vi "Update States.vi"(8 "error in (no error)":errorcluster, 11 "ATM Controller in":refnum<class "ATM Controller.lvclass">) -> (0 "error out":errorcluster, 3 "ATM Controller out":refnum<class "ATM Controller.lvclass">)   [LabVIEW 2019, in "ATM Controller.lvlib" / "ATM Controller.lvclass"]
uses:
  ATM Controller.lvclass
  ATM Controller Messages/Set State Msg/Set State Msg.lvclass
  <vilib>/ActorFramework/Actor/Actor.lvclass
  State -Enum.ctl
  ATM Controller Messages/Set ATM Message Msg/Set ATM Message Msg.lvclass
  Message Name.ctl
  Simulated User Console Actor/Simulated User Console Actor Messages/Enable Card Reader Msg/Enable Card Reader Msg.lvclass
  Simulated User Console Actor/Simulated User Console Actor Messages/Enable Keypad Msg/Enable Keypad Msg.lvclass
  Simulated User Console Actor/Simulated User Console Actor Messages/Enable Transaction Msg/Enable Transaction Msg.lvclass
  Simulated Display Console Actor/Simulated Display Console Actor Messages/Write Card Read Msg/Write Card Read Msg.lvclass
  Simulated Display Console Actor/Simulated Display Console Actor Messages/Write Current Transaction Msg/Write Current Transaction Msg.lvclass
  Simulated Sensor Interface Actor/Simulated Sensor Interface Actor Messages/Disable All Controls Msg/Disable All Controls Msg.lvclass
  Simulated User Console Actor/Simulated User Console Actor Messages/Write Card Reader Msg/Write Card Reader Msg.lvclass
  Simulated User Console Actor/Simulated User Console Actor Messages/Disable Terminate Session Msg/Disable Terminate Session Msg.lvclass
  Simulated Configuration Database Actor/Configuration Database Actor Messages/Read Record Msg/Read Record Msg.lvclass
  <vilib>/ActorFramework/Message Enqueuer/Message Enqueuer.lvclass
  Simulated Configuration Database Actor/Configuration Database Actor Messages/Write Record Msg/Write Record Msg.lvclass
  ATM Controller Messages/Set Timeout Msg/Set Timeout Msg.lvclass
  Simulated User Console Actor/Simulated User Console Actor/Transactions -Cluster.ctl
  Simulated User Console Actor/Simulated User Console Actor/Simulated User Console Actor.lvclass
  Simulated User Console Actor/Simulated User Console Actor Messages/Enable New Transaction Msg/Enable New Transaction Msg.lvclass
  C:/Program Files (x86)/National Instruments/LabVIEW 2019/vi.lib/ActorFramework/Actor/Actor.lvclass
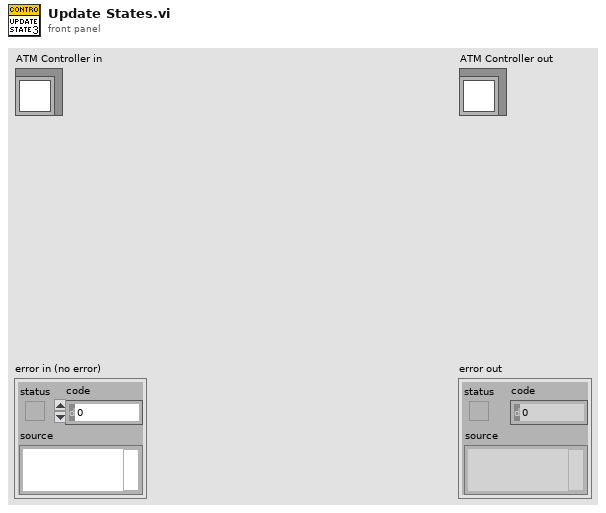
[diagram p1: front panel]
types:
  T1 = enum8{"Enabled", "Disabled", "Disabled and Grayed Out"}
  T2 = typedef "ATM Controller.lvlib/ATM Controller.lvclass/Message Name.ctl" = enum16{"Welcome", "Login", "Idle", "Invalid Login", "Terminate Session", "Deposit", "Withdrawal", "Fast Cash $50", "Withdrawal Failed", "Balance Inquiry"}
  T3 = typedef "ATM Controller.lvlib/ATM Controller.lvclass/State -Enum.ctl" = enum16{"Inital", "Idle", "Login", "Balance Inquiry", "Deposit", "Withdrawal", "Fast Cash", "Terminate"}
  T4 = typedef "Configuration Database Actor.lvlib/Configuration Database Actor.lvclass/Records -cluster.ctl" = cluster{"Account Number":i32, "First Name":string, "Last Name":string, "Balance":i32}
  T5 = typedef "Simulated User Console Actor.lvlib/Simulated User Console Actor.lvclass/Transactions -Cluster.ctl" = cluster{"Balance Inquiry":bool, "Deposit":bool, "Withdrawal":bool, "Fast Cash $50":bool, "New Transaction":bool, "Terminate Session":bool}
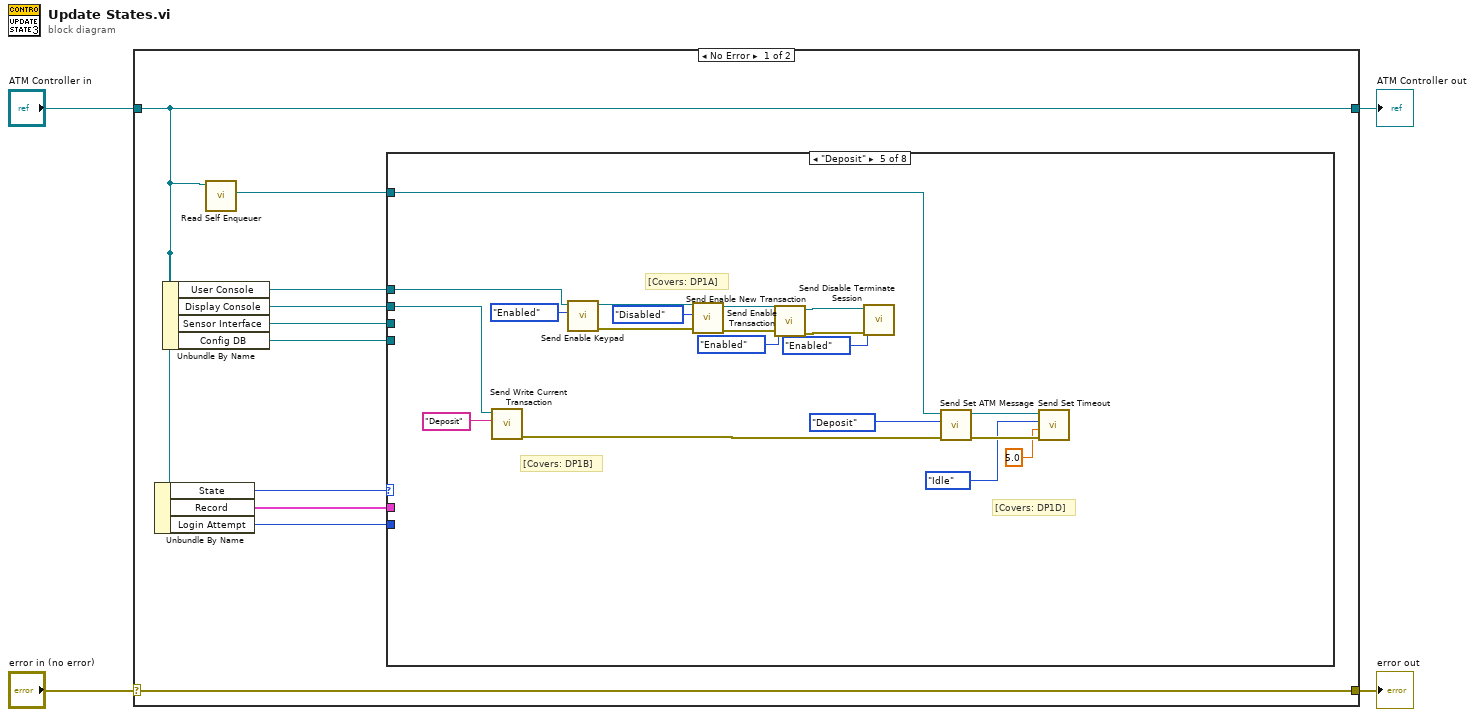
[diagram p0: block diagram]
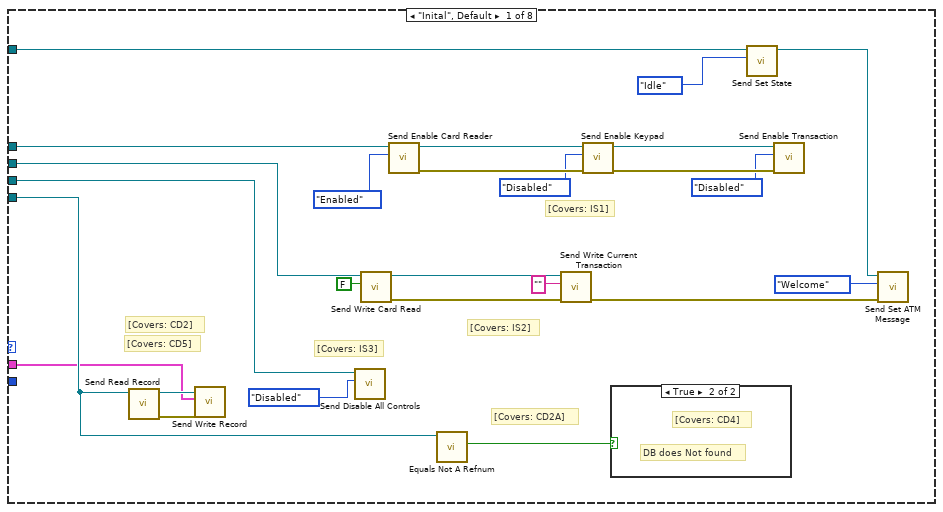
[diagram p2: hidden frame]
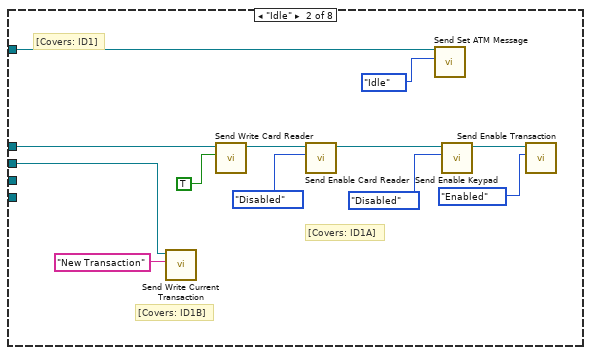
[diagram p4: hidden frame]
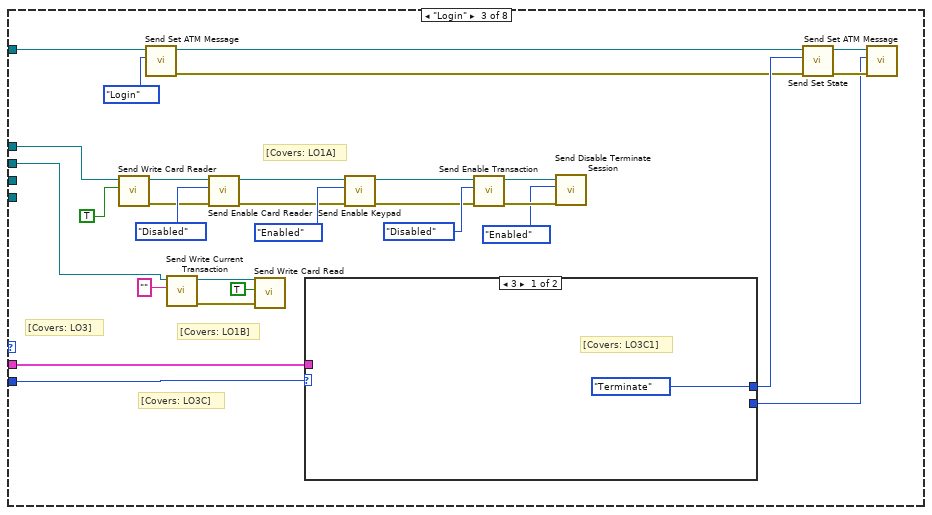
[diagram p5: hidden frame]
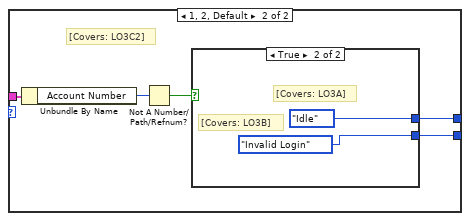
[diagram p6: hidden frame]
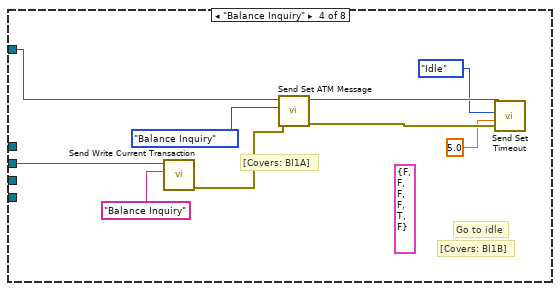
[diagram p8: hidden frame]
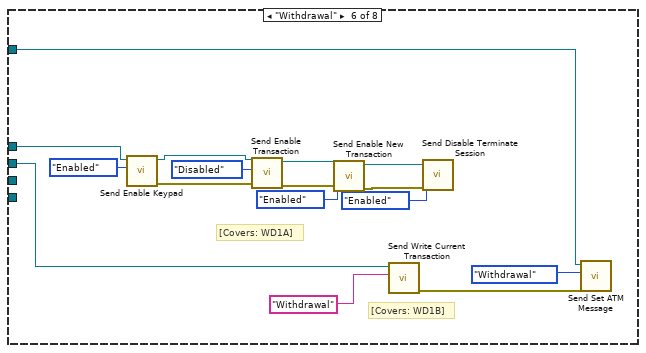
[diagram p9: hidden frame]
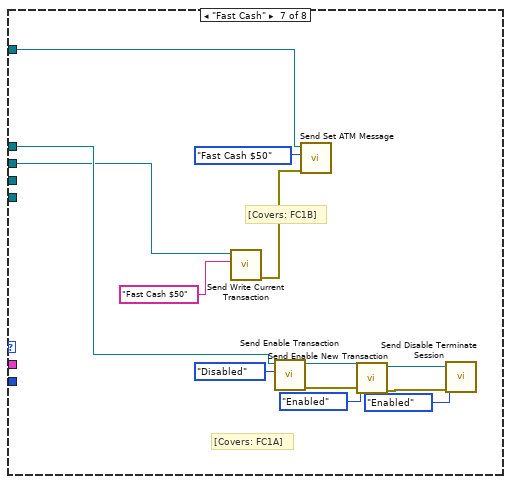
[diagram p10: hidden frame]
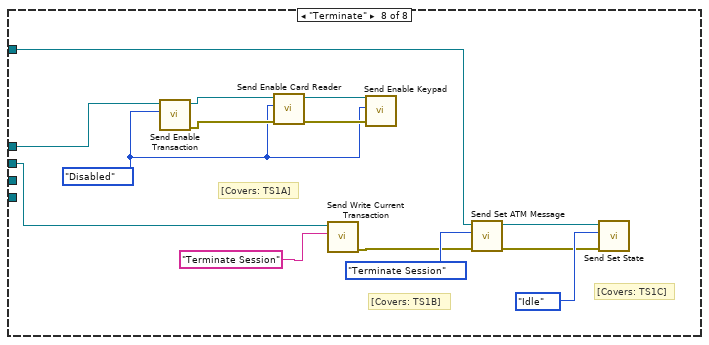
[diagram p11: hidden frame]
diagram:
  n1 = case shown="No Error" "error in (no error)" {
    selector: "error in (no error)" -> [w14 w162]
    tunnel: [w14 w162] -> w3
    tunnel: [w5 w161] -> w1
    tunnel: "ATM Controller in" -> [w5 w161]
    frame No Error {
      n2 = Unbundle By Name(w5) -> ("State"=w13:T3, "Record"=w7:T4, "Login Attempt"=w6:u8)
      n3 = Unbundle By Name(w5) -> ("User Console"=w11:refnum<class "Message Enqueuer.lvclass">, "Display Console"=w10:refnum<class "Message Enqueuer.lvclass">, "Sensor Interface"=w9:refnum<class "Message Enqueuer.lvclass">, "Config DB"=w8:refnum<class "Message Enqueuer.lvclass">)
      n4 = call <vilib>:"Read Self Enqueuer.vi"("Actor"=w5) -> ("Self Enqueuer"=w12:refnum<class "Message Enqueuer.lvclass">)  [unwired: 10 in]
      n5 = case shown="\"Deposit\"" w13 {
        tunnel: w12 -> [w39 w51 w58 w97 w117 w133 w145 w160]
        tunnel: w11 -> [w37 w42 w70 _ w111 w124 w137 w150]
        tunnel: w10 -> [w27 w40 w61 w95 w103 w119 w136 w149]
        tunnel: w9 -> [w21 _ _ _ _ _ _ _]
        tunnel: w8 -> [w18 _ _ _ _ _ _ _]
        tunnel: w7 -> [w15 _ w60 _ _ _ _ _]
        tunnel: w6 -> [_ _ w52 _ _ _ _ _]
        frame "Inital", Default {
          # "[Covers: CD5]"
          # "[Covers: CD2A]"
          # "[Covers: CD2]"
          # "[Covers: IS3]"
          # "[Covers: IS2]"
          # "[Covers: IS1]"
          n6 = call "Send Read Record.vi"("Message Enqueuer"=w18) -> ("error out"=w17:errorcluster, "Message Enqueuer out"=w16:refnum<class "Message Enqueuer.lvclass">)  [unwired: 9 in]
          n7 = call "Send Write Record.vi"("error in (no error)"=w17, "Record"=w15, "Message Enqueuer"=w16) -> ()  [unwired: 7 in, 2 out]
          n8 = call "Send Disable All Controls.vi"("Disabled"=T1."Disabled", "Message Enqueuer"=w21) -> ()  [unwired: 8 in, 2 out]
          n9 = call "Send Write Card Read.vi"("Card Read"=FALSE, "Message Enqueuer"=w27) -> ("error out"=w28:errorcluster, "Message Enqueuer out"=w29:refnum<class "Message Enqueuer.lvclass">)  [unwired: 8 in]
          n10 = call "Send Enable Card Reader.vi"("Disabled"=T1."Enabled", "Message Enqueuer"=w37) -> ("error out"=w34:errorcluster, "Message Enqueuer out"=w36:refnum<class "Message Enqueuer.lvclass">)  [unwired: 8 in]
          n11 = call <vilib>:"Equals Not A Refnum.vi"("Message Enqueuer"=w18) -> ("Not a refnum?"=w19:bool)  [unwired: 10 in]
          n12 = call "Send Write Current Transaction.vi"("error in (no error)"=w28, "Current Transaction"="", "Message Enqueuer"=w29) -> ("error out"=w24:errorcluster)  [unwired: 7 in, 1 out]
          n13 = call "Send Enable Keypad.vi"("error in (no error)"=w34, "Disabled"=T1."Disabled", "Message Enqueuer"=w36) -> ("error out"=w33:errorcluster, "Message Enqueuer out"=w35:refnum<class "Message Enqueuer.lvclass">)  [unwired: 7 in]
          n14 = case shown="True" w19 {
            frame False {
            }
            frame True {
              # "DB does Not found"
              # "[Covers: CD4]"
            }
          }
          n15 = call "Send Set State.vi"("State"=State_-Enum."Idle", "Message Enqueuer"=w39) -> ("Message Enqueuer out"=w22:refnum<class "Message Enqueuer.lvclass">)  [unwired: 8 in, 1 out]
          n16 = call "Send Enable Transaction.vi"("error in (no error)"=w33, "Disabled"=T1."Disabled", "Message Enqueuer"=w35) -> ()  [unwired: 7 in, 2 out]
          n17 = call "Send Set ATM Message.vi"("error in (no error)"=w24, "Message Name"=Message_Name."Welcome", "Message Enqueuer"=w22) -> ()  [unwired: 7 in, 2 out]
        }
        frame "Idle" {
          # "[Covers: ID1B]"
          # "[Covers: ID1A]"
          # "[Covers: ID1]"
          n18 = call "Send Write Current Transaction.vi"("Current Transaction"="New Transaction" ("Value"), "Message Enqueuer"=w40) -> ()  [unwired: 8 in, 2 out]
          n19 = call "Send Write Card Reader.vi"("Card Reader"=TRUE, "Message Enqueuer"=w42) -> ("Message Enqueuer out"=w44:refnum<class "Message Enqueuer.lvclass">)  [unwired: 8 in, 1 out]
          n20 = call "Send Enable Card Reader.vi"("Disabled"=T1."Disabled", "Message Enqueuer"=w44) -> ("Message Enqueuer out"=w46:refnum<class "Message Enqueuer.lvclass">)  [unwired: 8 in, 1 out]
          n21 = call "Send Set ATM Message.vi"("Message Name"=Message_Name."Idle", "Message Enqueuer"=w51) -> ()  [unwired: 8 in, 2 out]
          n22 = call "Send Enable Keypad.vi"("Disabled"=T1."Disabled", "Message Enqueuer"=w46) -> ("Message Enqueuer out"=w48:refnum<class "Message Enqueuer.lvclass">)  [unwired: 8 in, 1 out]
          n23 = call "Send Enable Transaction.vi"("Disabled"=T1."Enabled", "Message Enqueuer"=w48) -> ()  [unwired: 8 in, 2 out]
        }
        frame "Login" {
          # "[Covers: LO3C]"
          # "[Covers: LO3]"
          # "[Covers: LO1A]"
          # "[Covers: LO1B]"
          n24 = call "Send Write Card Reader.vi"("Card Reader"=TRUE, "Message Enqueuer"=w70) -> ("error out"=w73:errorcluster, "Message Enqueuer out"=w76:refnum<class "Message Enqueuer.lvclass">)  [unwired: 8 in]
          n25 = call "Send Set ATM Message.vi"("Message Name"=Message_Name."Login", "Message Enqueuer"=w58) -> ("error out"=w57:errorcluster, "Message Enqueuer out"=w56:refnum<class "Message Enqueuer.lvclass">)  [unwired: 8 in]
          n26 = call "Send Write Current Transaction.vi"("Current Transaction"="" ("Value"), "Message Enqueuer"=w61) -> ("error out"=w64:errorcluster, "Message Enqueuer out"=w65:refnum<class "Message Enqueuer.lvclass">)  [unwired: 8 in]
          n27 = call "Send Enable Card Reader.vi"("error in (no error)"=w73, "Disabled"=T1."Disabled", "Message Enqueuer"=w76) -> ("error out"=w72:errorcluster, "Message Enqueuer out"=w78:refnum<class "Message Enqueuer.lvclass">)  [unwired: 7 in]
          n28 = call "Send Write Card Read.vi"("error in (no error)"=w64, "Card Read"=TRUE, "Message Enqueuer"=w65) -> ()  [unwired: 7 in, 2 out]
          n29 = case shown="3" w52 {
            tunnel: w60 -> [_ w86]
            tunnel: [State_-Enum."Terminate" ("State") w83] -> w59
            tunnel: [_ w82] -> w53
            frame 3 {
              # "[Covers: LO3C1]"
            }
            frame 1, 2, Default {
              # "[Covers: LO3C2]"
              n30 = Unbundle By Name(w86) -> ("Account Number"=w85:i32)
              n31 = Not A Number/Path/Refnum?(number/path/refnum=w85) -> (NaN/Path/Refnum?=w84:bool)
              n32 = case shown="True" w84 {
                tunnel: [_ State_-Enum."Idle" ("State")] -> w83
                tunnel: [_ Message_Name."Invalid Login" ("Message Name")] -> w82
                frame False {
                }
                frame True {
                  # "[Covers: LO3B]"
                  # "[Covers: LO3A]"
                }
              }
            }
          }
          n33 = call "Send Enable Keypad.vi"("error in (no error)"=w72, "Disabled"=T1."Enabled", "Message Enqueuer"=w78) -> ("error out"=w71:errorcluster, "Message Enqueuer out"=w74:refnum<class "Message Enqueuer.lvclass">)  [unwired: 7 in]
          n34 = call "Send Enable Transaction.vi"("error in (no error)"=w71, "Disabled"=T1."Disabled", "Message Enqueuer"=w74) -> ("error out"=w68:errorcluster, "Message Enqueuer out"=w69:refnum<class "Message Enqueuer.lvclass">)  [unwired: 7 in]
          n35 = call "Send Disable Terminate Session.vi"("error in (no error)"=w68, "Disabled"=T1."Enabled", "Message Enqueuer"=w69) -> ()  [unwired: 7 in, 2 out]
          n36 = call "Send Set State.vi"("error in (no error)"=w57, "State"=w59, "Message Enqueuer"=w56) -> ("error out"=w55:errorcluster, "Message Enqueuer out"=w54:refnum<class "Message Enqueuer.lvclass">)  [unwired: 7 in]
          n37 = call "Send Set ATM Message.vi"("error in (no error)"=w55, "Message Name"=w53, "Message Enqueuer"=w54) -> ()  [unwired: 7 in, 2 out]
        }
        frame "Balance Inquiry" {
          (unwired) T5 {"Balance Inquiry"=FALSE, "Deposit"=FALSE, "Withdrawal"=FALSE, "Fast Cash $50"=FALSE, "New Transaction"=TRUE, "Terminate Session"=FALSE} ("Transactions")
          # "Go to idle"
          # "[Covers: BI1B]"
          # "[Covers: BI1A]"
          n38 = call "Send Write Current Transaction.vi"("Current Transaction"="Balance Inquiry" ("Value"), "Message Enqueuer"=w95) -> ("error out"=w93:errorcluster)  [unwired: 8 in, 1 out]
          n39 = call "Send Set ATM Message.vi"("error in (no error)"=w93, "Message Name"=Message_Name."Balance Inquiry", "Message Enqueuer"=w97) -> ("error out"=w92:errorcluster, "Message Enqueuer out"=w91:refnum<class "Message Enqueuer.lvclass">)  [unwired: 7 in]
          n40 = call "Send Set Timeout.vi"("error in (no error)"=w92, "Target Time"=5.0, "State"=State_-Enum."Idle", "Message Enqueuer"=w91) -> ()  [unwired: 6 in, 2 out]
        }
        frame "Deposit" {
          # "[Covers: DP1D]"
          # "[Covers: DP1B]"
          # "[Covers: DP1A]"
          n41 = call "Send Write Current Transaction.vi"("Current Transaction"="Deposit" ("Value"), "Message Enqueuer"=w103) -> ("error out"=w102:errorcluster)  [unwired: 8 in, 1 out]
          n42 = call "Send Enable Keypad.vi"("Disabled"=T1."Enabled", "Message Enqueuer"=w111) -> ("error out"=w114:errorcluster, "Message Enqueuer out"=w115:refnum<class "Message Enqueuer.lvclass">)  [unwired: 8 in]
          n43 = call "Send Enable Transaction.vi"("error in (no error)"=w114, "Disabled"=T1."Disabled", "Message Enqueuer"=w115) -> ("error out"=w109:errorcluster, "Message Enqueuer out"=w110:refnum<class "Message Enqueuer.lvclass">)  [unwired: 7 in]
          n44 = call "Send Enable New Transaction.vi"("error in (no error)"=w109, "Disabled"=T1."Enabled", "Message Enqueuer"=w110) -> ("error out"=w107:errorcluster, "Message Enqueuer out"=w106:refnum<class "Message Enqueuer.lvclass">)  [unwired: 7 in]
          n45 = call "Send Disable Terminate Session.vi"("error in (no error)"=w107, "Disabled"=T1."Enabled", "Message Enqueuer"=w106) -> ()  [unwired: 7 in, 2 out]
          n46 = call "Send Set ATM Message.vi"("error in (no error)"=w102, "Message Name"=Message_Name."Deposit", "Message Enqueuer"=w117) -> ("error out"=w100:errorcluster, "Message Enqueuer out"=w101:refnum<class "Message Enqueuer.lvclass">)  [unwired: 7 in]
          n47 = call "Send Set Timeout.vi"("error in (no error)"=w100, "Target Time"=5.0, "State"=State_-Enum."Idle", "Message Enqueuer"=w101) -> ()  [unwired: 6 in, 2 out]
        }
        frame "Withdrawal" {
          # "[Covers: WD1B]"
          # "[Covers: WD1A]"
          n48 = call "Send Enable Keypad.vi"("Disabled"=T1."Enabled", "Message Enqueuer"=w124) -> ("error out"=w131:errorcluster, "Message Enqueuer out"=w123:refnum<class "Message Enqueuer.lvclass">)  [unwired: 8 in]
          n49 = call "Send Enable Transaction.vi"("error in (no error)"=w131, "Disabled"=T1."Disabled", "Message Enqueuer"=w123) -> ("error out"=w128:errorcluster, "Message Enqueuer out"=w122:refnum<class "Message Enqueuer.lvclass">)  [unwired: 7 in]
          n50 = call "Send Enable New Transaction.vi"("error in (no error)"=w128, "Disabled"=T1."Enabled", "Message Enqueuer"=w122) -> ("error out"=w126:errorcluster, "Message Enqueuer out"=w121:refnum<class "Message Enqueuer.lvclass">)  [unwired: 7 in]
          n51 = call "Send Write Current Transaction.vi"("Current Transaction"="Withdrawal" ("Value"), "Message Enqueuer"=w119) -> ("error out"=w118:errorcluster)  [unwired: 8 in, 1 out]
          n52 = call "Send Disable Terminate Session.vi"("error in (no error)"=w126, "Disabled"=T1."Enabled", "Message Enqueuer"=w121) -> ()  [unwired: 7 in, 2 out]
          n53 = call "Send Set ATM Message.vi"("error in (no error)"=w118, "Message Name"=Message_Name."Withdrawal", "Message Enqueuer"=w133) -> ()  [unwired: 7 in, 2 out]
        }
        frame "Fast Cash" {
          # "[Covers: FC1B]"
          # "[Covers: FC1A]"
          n54 = call "Send Write Current Transaction.vi"("Current Transaction"="Fast Cash $50" ("Value"), "Message Enqueuer"=w136) -> ("error out"=w135:errorcluster)  [unwired: 8 in, 1 out]
          n55 = call "Send Enable Transaction.vi"("Disabled"=T1."Disabled", "Message Enqueuer"=w137) -> ("error out"=w143:errorcluster, "Message Enqueuer out"=w139:refnum<class "Message Enqueuer.lvclass">)  [unwired: 8 in]
          n56 = call "Send Set ATM Message.vi"("error in (no error)"=w135, "Message Name"=Message_Name."Fast Cash $50", "Message Enqueuer"=w145) -> ()  [unwired: 7 in, 2 out]
          n57 = call "Send Enable New Transaction.vi"("error in (no error)"=w143, "Disabled"=T1."Enabled", "Message Enqueuer"=w139) -> ("error out"=w141:errorcluster, "Message Enqueuer out"=w138:refnum<class "Message Enqueuer.lvclass">)  [unwired: 7 in]
          n58 = call "Send Disable Terminate Session.vi"("error in (no error)"=w141, "Disabled"=T1."Enabled", "Message Enqueuer"=w138) -> ()  [unwired: 7 in, 2 out]
        }
        frame "Terminate" {
          w151 = T1."Disabled" ("Disabled")
          # "[Covers: TS1C]"
          # "[Covers: TS1B]"
          # "[Covers: TS1A]"
          n59 = call "Send Enable Transaction.vi"("Disabled"=w151, "Message Enqueuer"=w150) -> ("error out"=w153:errorcluster, "Message Enqueuer out"=w155:refnum<class "Message Enqueuer.lvclass">)  [unwired: 8 in]
          n60 = call "Send Enable Card Reader.vi"("error in (no error)"=w153, "Disabled"=w151, "Message Enqueuer"=w155) -> ("error out"=w152:errorcluster, "Message Enqueuer out"=w154:refnum<class "Message Enqueuer.lvclass">)  [unwired: 7 in]
          n61 = call "Send Write Current Transaction.vi"("Current Transaction"="Terminate Session" ("Value"), "Message Enqueuer"=w149) -> ("error out"=w148:errorcluster)  [unwired: 8 in, 1 out]
          n62 = call "Send Enable Keypad.vi"("error in (no error)"=w152, "Disabled"=w151, "Message Enqueuer"=w154) -> ()  [unwired: 7 in, 2 out]
          n63 = call "Send Set ATM Message.vi"("error in (no error)"=w148, "Message Name"=Message_Name."Terminate Session", "Message Enqueuer"=w160) -> ("error out"=w156:errorcluster, "Message Enqueuer out"=w158:refnum<class "Message Enqueuer.lvclass">)  [unwired: 7 in]
          n64 = call "Send Set State.vi"("error in (no error)"=w156, "State"=State_-Enum."Idle", "Message Enqueuer"=w158) -> ()  [unwired: 7 in, 2 out]
        }
      }
    }
    frame Error {
    }
  }
  "error out" <- w3
  "ATM Controller out" <- w1
